vi "DCM Properties.vi"() -> ()   [LabVIEW 2016, in "DCM Shared.lvlib"]
uses:
  DCM Shared.lvlib
panel:
  in  "Tab Control":T1(tab)
  in  "Main.Password":string="Main.Password"
  in  "Main.Username":string="Main.Username"
  in  "Main.DCM Model":string="Main.DCM Model"
  in  "Main.Rate-Sys":string="Main.Rate-Sys"
  in  "Main.Rate-Cmd":string="Main.Rate-Cmd"
  in  "Main.Priority-Sys":string="Main.Priority-Sys"
  in  "Main.Priority-Cmd":string="Main.Priority-Cmd"
  in  "Main.CPU-Sys":string="Main.CPU-Sys"
  in  "Main.FPGA Resource":string="Main.FPGA Resource"
  in  "Main.IP Address":string="Main.IP Address"
  in  "Main.FPGA Location":string="Main.FPGA Location"
  in  "Main.Bitfile Path":string="Main.Bitfile Path"
  in  "Main.DCMCreated":string="Main.DCMCreated"
  in  "Main.Cam Captures":string="Main.Cam Captures"
  in  "Main.CompiledData":string="Main.CompiledData"
  in  "Main.CPU-Cmd":string="Main.CPU-Cmd"
  in  "Main.validBitfile":string="Main.validBitfile"
  in  "IP.bitfile name":string="IP.bitfile name"
  in  "Main.bitfile EPS version":string="Main.bitfile EPS version"
  in  "Main.Bitfile":string="Main.Bitfile"
  in  "Main.Device Address":string="Main.Device Address"
  in  "System.Settings":string="System.Settings"
  in  "System.State Indexes":string="System.State Indexes"
  in  "System.Status":string="System.Status"
  in  "Knock.Command Enabled":string="Knock.Command Enabled"
  in  "Knock.Settings":string="Knock.Settings"
  in  "EPTx.SignalSelect":string="EPTx.SignalSelect"
  in  "EPTx.Configuration":string="EPTx.Configuration"
  in  "DI-A.PumpCommand":string="DI-A.PumpCommand"
  in  "DI-A.Sync Pump Enabled":string="DI-A.Sync Pump Enabled"
  in  "DI-A.FaultIndexes":string="DI-A.FaultIndexes"
  in  "DI-A.Command Enabled":string="DI-A.Command Enabled"
  in  "DI-A.CommandArrayIndexes":string="DI-A.CommandArrayIndexes"
  in  "DI-A.PhaseArrays":string="DI-A.PhaseArrays"
  in  "DI-A.PumpPhaseArray":string="DI-A.PumpPhaseArray"
  in  "DI-A.CommandArray":string="DI-A.CommandArray"
  in  "DI-A.Configuration":string="DI-A.Configuration"
  in  "DI-A.Simulation":string="DI-A.Simulation"
  in  "DI-B.PumpCommand":string="DI-B.PumpCommand"
  in  "DI-B.Sync Pump Enabled":string="DI-B.Sync Pump Enabled"
  in  "DI-B.FaultIndexes":string="DI-B.FaultIndexes"
  in  "DI-B.Command Enabled":string="DI-B.Command Enabled"
  in  "DI-B.CommandArrayIndexes":string="DI-B.CommandArrayIndexes"
  in  "DI-B.PhaseArrays":string="DI-B.PhaseArrays"
  in  "DI-B.PumpPhaseArray":string="DI-B.PumpPhaseArray"
  in  "DI-B.CommandArray":string="DI-B.CommandArray"
  in  "DI-B.Configuration":string="DI-B.Configuration"
  in  "DI-B.Simulation":string="DI-B.Simulation"
  in  "DiffIO.Filters":string="DiffIO.Filters"
  in  "DiffIO.Channel Names":string="DiffIO.Channel Names"
  in  "DiffIO.Command Enabled":string="DiffIO.Command Enabled"
  in  "DiffIO.SetupIndexes":string="DiffIO.SetupIndexes"
  in  "DiffIO.ResultsIndexes":string="DiffIO.ResultsIndexes"
  in  "DiffIO.Setup":string="DiffIO.Setup"
  in  "DiffIO.Results":string="DiffIO.Results"
  in  "Aux.SerialIn2":string="Aux.SerialIn2"
  in  "Aux.SerialIn1":string="Aux.SerialIn1"
  in  "Aux.Filters":string="Aux.Filters"
  in  "Aux.Channel Names":string="Aux.Channel Names"
  in  "ESTTL.Channel Names":string="ESTTL.Channel Names"
  in  "ESTTL.Command Enabled":string="ESTTL.Command Enabled"
  in  "ESTTL.SetupIndexes":string="ESTTL.SetupIndexes"
  in  "ESTTL.Setup":string="ESTTL.Setup"
  in  "VR-Hall.Arming Threshold":string="VR-Hall.Arming Threshold"
  in  "VR-Hall.Mode Select":string="VR-Hall.Mode Select"
  in  "HH.Channel Names":string="HH.Channel Names"
  in  "HH.Status Indexes":string="HH.Status Indexes"
  in  "HH.Config Indexes":string="HH.Config Indexes"
  in  "HH.Command Enabled":string="HH.Command Enabled"
  in  "HH.Config":string="HH.Config"
  in  "HH.Command Indexes":string="HH.Command Indexes"
  in  "HH.Command":string="HH.Command"
  in  "Skipfire.Channel Names":string="Skipfire.Channel Names"
  in  "Skipfire.Command Enabled":string="Skipfire.Command Enabled"
  in  "Skipfire.SetupIndexes":string="Skipfire.SetupIndexes"
  in  "Skipfire.Setup":string="Skipfire.Setup"
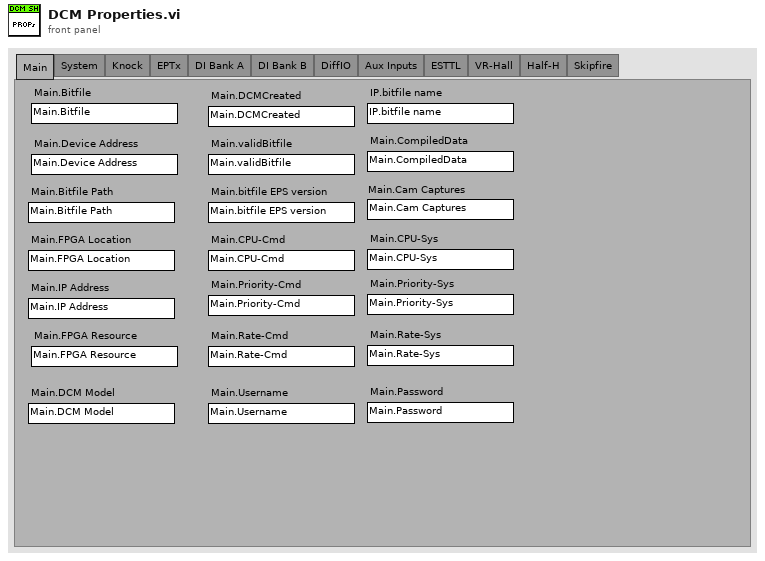
[diagram p1: front panel]
types:
  T1 = enum32{"Main", "System", "Knock", "EPTx", "DI Bank A", "DI Bank B", "DiffIO", "Aux Inputs", "ESTTL", "VR-Hall", "Half-H", "Skipfire"}
diagram:
